vi "Main.vi"(11 "Module Admin":refnum<class "Delacor_lib_QMH_Cloneable Module Admin.lvclass">) -> ()   [LabVIEW 2025, in "My Cloneable Module.lvlib"]
doc: "This template is based off of the Queued Message Handler design pattern and the Queued Message Handler project template that ships with LabVIEW.\n\nThe main difference is that the queue is private to this module and communication between modules is performed via Broadcast and Request events.\n\nRequest events are wrapped in public API methods and are handled in the Event Handling Loop (EHL) of this VI. Any module can register for Broadcast events sent by this module. The EHL generates messages based on user interface actions.\n\nThe Message Handling Loop (MHL) processes messages generated by the EHL, or by other messages. The messages are string values, so new messages can be added easily to the Message Cases case structure in the MHL. Each message cluster can also provide an optional value for Message Data, which is a variant that can be converted to whatever message-specific data is required.\n_____\nBased on DQMH Dev Tools: Project Template 7.1.0.1503."
uses:
  My Cloneable Module.lvlib
  <vilib>/Delacor/Delacor QMH/Libraries/Cloneable Module Admin_class/Delacor_lib_QMH_Cloneable Module Admin.lvclass
  C:/Program Files (x86)/National Instruments/LabVIEW 2025/vi.lib/Delacor/Delacor QMH/Libraries/Module Admin_class/Delacor_lib_QMH_Module Admin.lvclass
  Module Data--cluster.ctl
  Do Something Argument--cluster.ctl
  <vilib>/Delacor/Delacor QMH/Libraries/Cloneable Module Admin_class/Delacor_lib_QMH_Cloneable Module Admin.lvclass/Delacor_lib_QMH_Cloneable Module Admin.ctl
  <vilib>/Delacor/Delacor QMH/Libraries/Message Queue_class/Delacor_lib_QMH_Message Queue.lvclass/Delacor_lib_QMH_Message Queue.ctl
  Do Something Else Argument--cluster.ctl
  Do Something Else and Wait for Reply Argument--cluster.ctl
  Do Something Else and Wait (Reply Payload)--cluster.ctl
  Stop Argument--cluster.ctl
  <vilib>/Delacor/Delacor QMH/Libraries/Module Admin_class/Delacor_lib_QMH_Module Admin.lvclass/Delacor_lib_QMH_Module Admin.ctl
  <vilib>/Utility/miscctls.llb/LVPointTypeDef.ctl
  <vilib>/Delacor/Delacor QMH/Libraries/Message Queue_class/Delacor_lib_QMH_Enqueue Message (Single).vi
  <vilib>/Delacor/Delacor QMH/Libraries/Cloneable Module Admin_class/Delacor_lib_QMH_Get Module ID.vi
  <vilib>/Delacor/Delacor QMH/Libraries/Module Admin_class/Delacor_lib_QMH_Get External Launch.vi
  <vilib>/Delacor/Delacor QMH/Libraries/Message Queue_class/Delacor_lib_QMH_Message Queue.lvclass
panel:
  out "error out":errorcluster
  out "X":dbl
  out "Status":string
  in  "Simulate EHL Error":bool
  in  "Simulate MHL Error":bool
  in  "Do Something Else <Replace Me>":bool
  in  "Do Something <Replace Me>":bool
  # "These controls have associated \"Value Changed\" events configured in the Event Structure on the diagram.\n\nReplace them (and reconfigure the Event Structure) with the controls you need for your application. \n\nOther processes communicate with this Module via its Public API (wrappers for its Request Events).\n\nThis Module communicates with other processes via its Broadcast Events.\nAny process that wants to receive these messages can register for this module's Broadcast events."
  # "This template is for the DQMH framework. See the block diagram for more information on how to use this template."
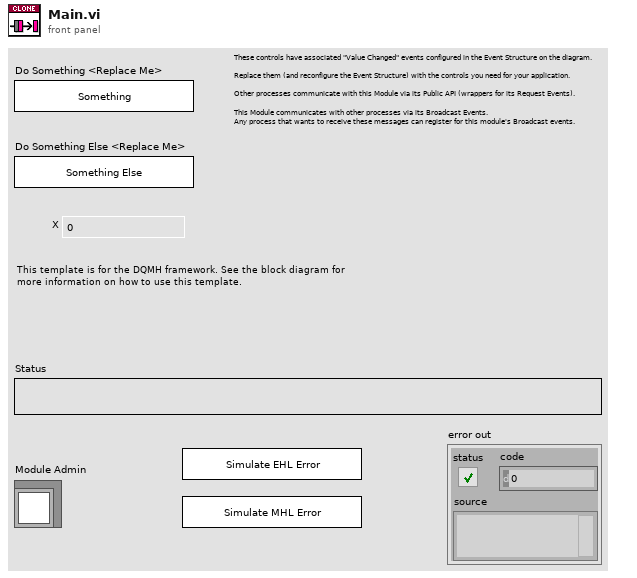
[diagram p1: front panel]
types:
  T1 = typedef "My Cloneable Module.lvlib/Request Events--cluster.ctl" = cluster{"Stop Module":refnum<user-event>, "Do Something":refnum<user-event>, "Do Something Else":refnum<user-event>, "Do Something Else and Wait for Reply":refnum<user-event>, "Show Panel":refnum<user-event>, "Hide Panel":refnum<user-event>, "Show Diagram":refnum<user-event>, "Get Module Execution Status":refnum<user-event>}
  T2 = typedef "My Cloneable Module.lvlib/Module Data--cluster.ctl" = cluster{"Status":string}
  T3 = typedef "My Cloneable Module.lvlib/Do Something Argument--cluster.ctl" = cluster{"Module ID":i32, "Do Something Msg":string}
  T4 = typedef "My Cloneable Module.lvlib/Do Something Else Argument--cluster.ctl" = cluster{"Module ID":i32, "Do Something Else Msg":string, "X":dbl}
  T5 = typedef "My Cloneable Module.lvlib/Do Something Else and Wait for Reply Argument--cluster.ctl" = cluster{"Module ID":i32, "Do Something Else Msg":string, "X":dbl, "Wait Notifier":refnum<notifier>, "wait for reply":bool}
  T6 = enum32{"invalid lock state", "Not Locked", "Locked (No Password)", "Password-protected"}
  T7 = typedef "My Cloneable Module.lvlib/Stop Argument--cluster.ctl" = cluster{"Module ID":i32, "Origin":string, "Exit via Stop Module Req?":bool, "Wait for Module to stop?":bool}
  T8 = typedef "LVPointTypeDef.ctl" = cluster{"Horizontal":i16, "Vertical":i16}
  T9 = enum32{"Invalid", "Standard", "Closed", "Hidden", "Minimized", "Maximized"}
  T10 = typedef "My Cloneable Module.lvlib/Do Something Else and Wait (Reply Payload)--cluster.ctl" = cluster{"Value":dbl, "error":errorcluster, "Module ID":i32}
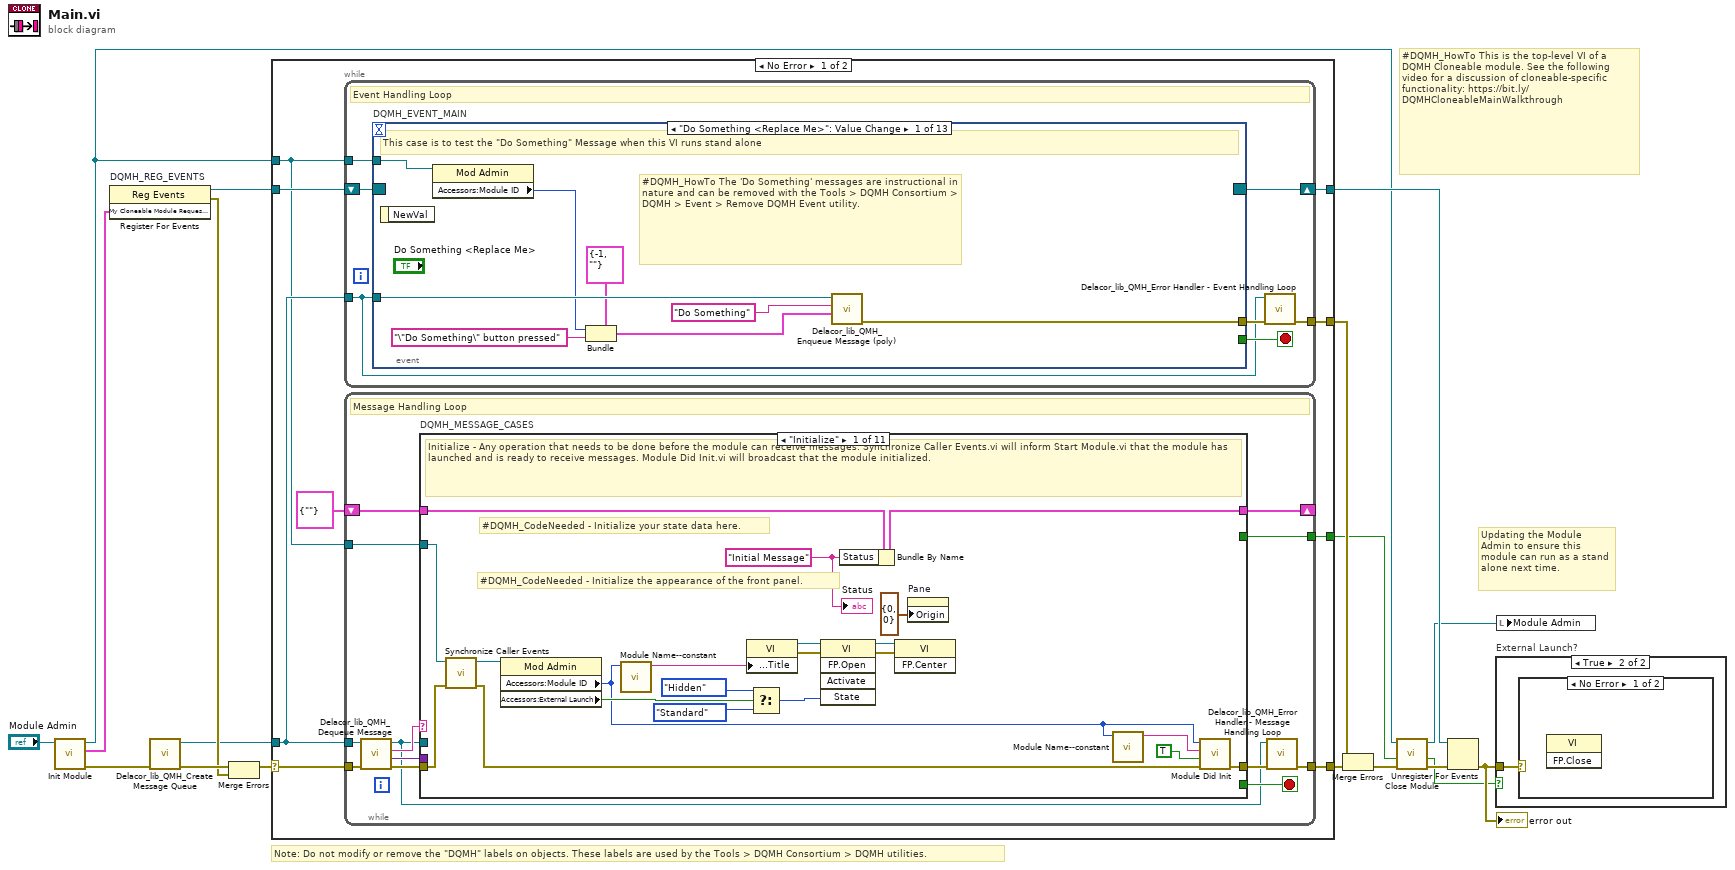
[diagram p0: block diagram]
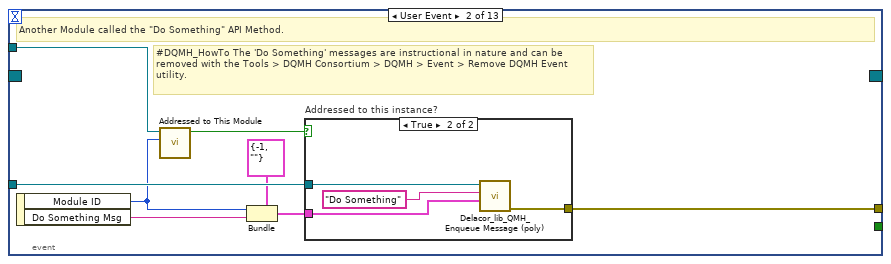
[diagram p2: hidden frame]
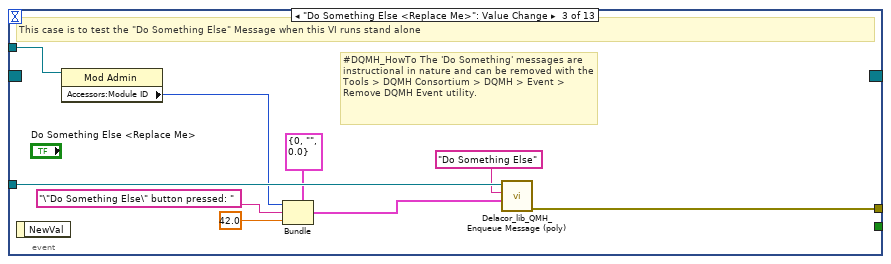
[diagram p4: hidden frame]
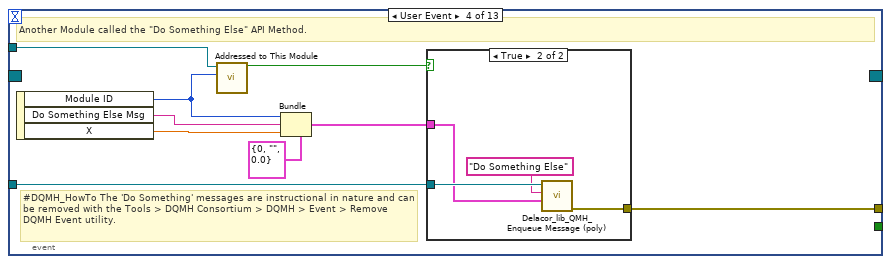
[diagram p5: hidden frame]
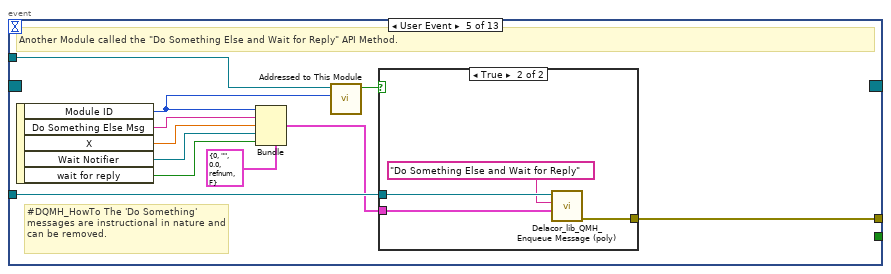
[diagram p7: hidden frame]
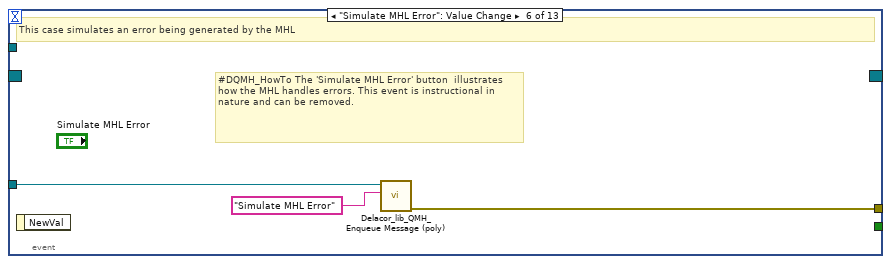
[diagram p9: hidden frame]
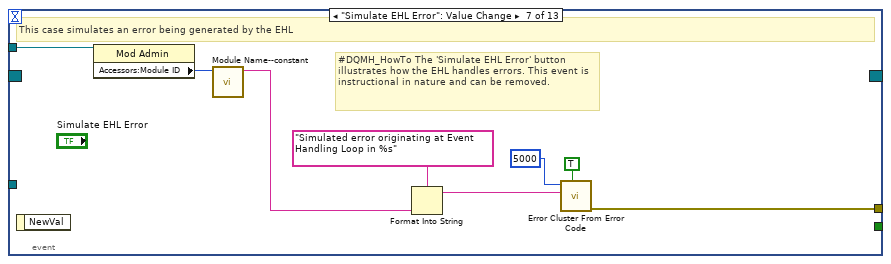
[diagram p10: hidden frame]
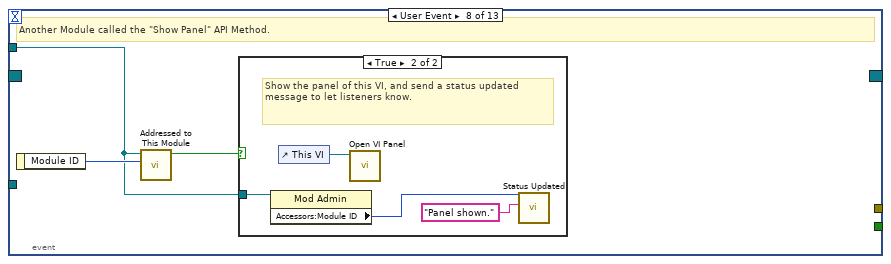
[diagram p11: hidden frame]
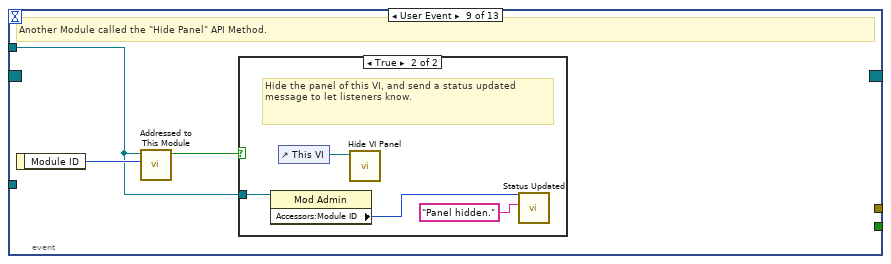
[diagram p13: hidden frame]
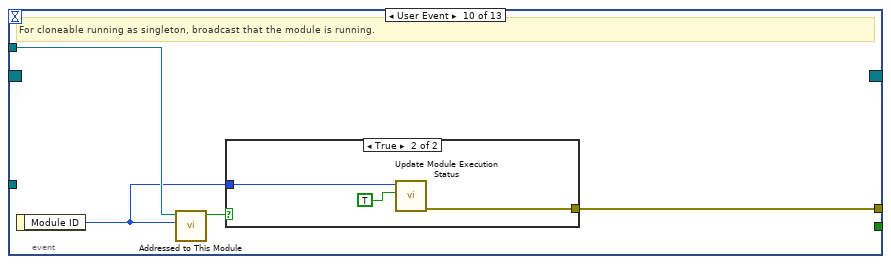
[diagram p15: hidden frame]
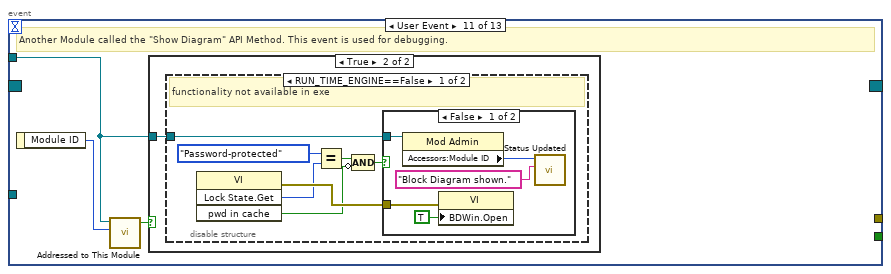
[diagram p17: hidden frame]
diagram:
  # "#DQMH_HowTo This is the top-level VI of a DQMH Cloneable module. See the following video for a discussion of cloneable-specific functionality: https://bit.ly/DQMHCloneableMainWalkthrough"
  # "Note: Do not modify or remove the \"DQMH\" labels on objects. These labels are used by the Tools > DQMH Consortium > DQMH utilities."
  # "Updating the Module Admin to ensure this module can run as a stand alone next time."
  n1 = call "Init Module.vi"("Cloneable Module Admin in"="Module Admin") -> ("error out"=w15:errorcluster, "My Cloneable Module Request Events"=w7:T1, "Cloneable Module Admin out"=w4:refnum<class "Delacor_lib_QMH_Cloneable Module Admin.lvclass">)  [unwired: 8 in]
  n2 = register-events "DQMH_REG_EVENTS"(w7) -> (reference out=w8:refnum<event-registration>, error out=w10:errorcluster)  [unwired: 2 in]
  n3 = call <vilib>:"Delacor_lib_QMH_Create Message Queue.vi"("error in"=w15) -> ("error out"=w12:errorcluster, "Message Queue"=w6:refnum<class "Delacor_lib_QMH_Message Queue.lvclass">)  [unwired: 9 in]
  n4 = Merge Errors(w12, w10) -> (w11:errorcluster)
  n5 = case shown="No Error" w11 {
    selector: w11 -> [w25 w336]
    tunnel: [w27 w335] -> w16
    tunnel: [w24 w334] -> w9
    tunnel: w8 -> [w22 w334]
    tunnel: w6 -> [w21 w327]
    tunnel: [w26 _] -> w17
    tunnel: w4 -> [w20 w330]
    tunnel: [w19 _] -> w2
    frame No Error {
      n6 = while {
        tunnel: w21 -> [w28]
        shift-right: [w31] -> w24
        shift-left: w22 -> [w32]
        tunnel: [w33] -> w26
        tunnel: w20 -> [w29]
        stop <- w30 stop-if-true
        # "Event Handling Loop"
        n7 = event "DQMH_EVENT_MAIN" shown="[0] \"Do Something <Replace Me>\": Value Change" {
          selector: w32 -> [_ _ _ _ _ _ _ _ _ _ _ _ _]
          dyn-events: [_ _ _ _ _ _ _ _ _ _ _ _ _] -> w31
          timeout: _ -> [_ _ _ _ _ _ _ _ _ _ _ _ _]
          tunnel: [_ _ _ _ _ _ _ _ _ _ _ w143 _] -> w30
          tunnel: w28 -> [w41 w49 w62 w71 w86 w93 _ _ _ _ _ w146 w163]
          tunnel: [w42 w50 w63 w72 w87 w94 w102 _ _ w120 _ w147 w166] -> w34
          tunnel: w29 -> [w37 w47 w56 w69 w84 _ w101 w103 w110 w118 w124 w145 w164]
          event "Do Something <Replace Me>": Value Change {
            # "#DQMH_HowTo The 'Do Something' messages are instructional in nature and can be removed with the Tools > DQMH Consortium > DQMH > Event > Remove DQMH Event utility."
            # "This case is to test the \"Do Something\" Message when this VI runs stand alone"
            n8 = event-data() -> ()  [unwired: 1 in, 1 out]
            n9 = property on="Property Node" class="Mod Admin"(reference=w37) -> ("Accessors:Module ID"=w36:i32)  [unwired: 1 in, 2 out]
            n10 = Bundle(cluster=T3 {"Module ID"=-1, "Do Something Msg"=""} ("Do Something Argument"), "Module ID"=w36, "Do Something Msg"="\"Do Something\" button pressed" ("\"Do Something\" button pressed")) -> (w39:T3)
            n11 = call-poly <vilib>:"Delacor_lib_QMH_Enqueue Message (poly).vi"("Message Data"=w39, "Message"="Do Something", "Message Queue in"=w41) -> ("error out"=w42:errorcluster)  [unwired: 7 in, 1 out]
          }
          event User Event {
            # "#DQMH_HowTo The 'Do Something' messages are instructional in nature and can be removed with the Tools > DQMH Consortium > DQMH > Event > Remove DQMH Event utility."
            # "Another Module called the \"Do Something\" API Method."
            n12 = event-data() -> ("Module ID"=w44:i32, "Do Something Msg"=w43:string)  [unwired: 1 in]
            n13 = call "Addressed to This Module.vi"("Module ID from Argument"=w44, "Module Admin"=w47) -> ("Addressed to this instance?"=w48:bool)  [unwired: 8 in, 1 out]
            n14 = Bundle(cluster=T3 {"Module ID"=-1, "Do Something Msg"=""} ("Do Something Argument"), "Module ID"=w44, "Do Something Msg"=w43) -> (w46:T3)
            n15 = case "Addressed to this instance?" shown="True" w48 {
              tunnel: w49 -> [_ w53]
              tunnel: [_ w54] -> w50
              tunnel: w46 -> [_ w51]
              frame False {
                # "Do nothing"
              }
              frame True {
                n16 = call-poly <vilib>:"Delacor_lib_QMH_Enqueue Message (poly).vi"("Message Data"=w51, "Message"="Do Something", "Message Queue in"=w53) -> ("error out"=w54:errorcluster)  [unwired: 7 in, 1 out]
              }
            }
          }
          event "Do Something Else <Replace Me>": Value Change {
            # "#DQMH_HowTo The 'Do Something' messages are instructional in nature and can be removed with the Tools > DQMH Consortium > DQMH > Event > Remove DQMH Event utility."
            # "This case is to test the \"Do Something Else\" Message when this VI runs stand alone"
            n17 = event-data() -> ()  [unwired: 1 in, 1 out]
            n18 = property on="Property Node" class="Mod Admin"(reference=w56) -> ("Accessors:Module ID"=w55:i32)  [unwired: 1 in, 2 out]
            n19 = Bundle(cluster=T4 {"Module ID"=0, "Do Something Else Msg"="", "X"=0.0} ("Do Something Else Argument"), "Module ID"=w55, "Do Something Else Msg"="\"Do Something Else\" button pressed: " ("\"Do Something Else\" button pressed"), "X"=42.0) -> (w59:T4)
            n20 = call-poly <vilib>:"Delacor_lib_QMH_Enqueue Message (poly).vi"("Message Data"=w59, "Message"="Do Something Else", "Message Queue in"=w62) -> ("error out"=w63:errorcluster)  [unwired: 7 in, 1 out]
          }
          event User Event {
            # "#DQMH_HowTo The 'Do Something' messages are instructional in nature and can be removed with the Tools > DQMH Consortium > DQMH > Event > Remove DQMH Event utility."
            # "Another Module called the \"Do Something Else\" API Method."
            n21 = event-data() -> ("Module ID"=w64:i32, "Do Something Else Msg"=w65:string, "X"=w67:dbl)  [unwired: 1 in]
            n22 = call "Addressed to This Module.vi"("Module ID from Argument"=w64, "Module Admin"=w69) -> ("Addressed to this instance?"=w70:bool)  [unwired: 8 in, 1 out]
            n23 = Bundle(cluster=T4 {"Module ID"=0, "Do Something Else Msg"="", "X"=0.0} ("Do Something Else Argument"), "Module ID"=w64, "Do Something Else Msg"=w65, "X"=w67) -> (w66:T4)
            n24 = case shown="True" w70 {
              tunnel: w71 -> [_ w75]
              tunnel: [_ w76] -> w72
              tunnel: w66 -> [_ w73]
              frame False {
              }
              frame True {
                n25 = call-poly <vilib>:"Delacor_lib_QMH_Enqueue Message (poly).vi"("Message Data"=w73, "Message"="Do Something Else", "Message Queue in"=w75) -> ("error out"=w76:errorcluster)  [unwired: 7 in, 1 out]
              }
            }
          }
          event User Event {
            # "#DQMH_HowTo The 'Do Something' messages are instructional in nature and can be removed."
            # "Another Module called the \"Do Something Else and Wait for Reply\" API Method."
            n26 = event-data() -> ("Module ID"=w82:i32, "Do Something Else Msg"=w80:string, "X"=w79:dbl, "Wait Notifier"=w78:refnum<notifier>, "wait for reply"=w77:bool)  [unwired: 1 in]
            n27 = Bundle(cluster=T5 {"Module ID"=0, "Do Something Else Msg"="", "X"=0.0, "Wait Notifier"=refnum, "wait for reply"=FALSE} ("Do Something Else and Wait for Reply Argument"), "Module ID"=w82, "Do Something Else Msg"=w80, "X"=w79, "Wait Notifier"=w78, "wait for reply"=w77) -> (w81:T5)
            n28 = call "Addressed to This Module.vi"("Module ID from Argument"=w82, "Module Admin"=w84) -> ("Addressed to this instance?"=w85:bool)  [unwired: 8 in, 1 out]
            n29 = case shown="True" w85 {
              tunnel: [_ w91] -> w87
              tunnel: w86 -> [_ w90]
              tunnel: w81 -> [_ w88]
              frame False {
              }
              frame True {
                n30 = call-poly <vilib>:"Delacor_lib_QMH_Enqueue Message (poly).vi"("Message Data"=w88, "Message"="Do Something Else and Wait for Reply", "Message Queue in"=w90) -> ("error out"=w91:errorcluster)  [unwired: 7 in, 1 out]
              }
            }
          }
          event "Simulate MHL Error": Value Change {
            # "#DQMH_HowTo The 'Simulate MHL Error' button  illustrates how the MHL handles errors. This event is instructional in nature and can be removed."
            # "This case simulates an error being generated by the MHL"
            n31 = event-data() -> ()  [unwired: 1 in, 1 out]
            n32 = call-poly <vilib>:"Delacor_lib_QMH_Enqueue Message (poly).vi"("Message"="Simulate MHL Error", "Message Queue in"=w93) -> ("error out"=w94:errorcluster)  [unwired: 8 in, 1 out]
          }
          event "Simulate EHL Error": Value Change {
            # "#DQMH_HowTo The 'Simulate EHL Error' button  illustrates how the EHL handles errors. This event is instructional in nature and can be removed."
            # "This case simulates an error being generated by the EHL"
            n33 = event-data() -> ()  [unwired: 1 in, 1 out]
            n34 = property on="Property Node" class="Mod Admin"(reference=w101) -> ("Accessors:Module ID"=w100:i32)  [unwired: 1 in, 2 out]
            n35 = call "Module Name--constant.vi"("Module ID"=w100) -> ("Module Name"=w95:string)  [unwired: 10 in]
            n36 = Format Into String(format string="Simulated error originating at Event Handling Loop in %s", w95) -> (resulting string=w98:string)  [unwired: 2 in, 1 out]
            n37 = call <vilib>:"Error Cluster From Error Code.vi"("show call chain? (False)"=TRUE, "error message (\"\")"=w98, "error code (0)"=5000) -> ("error out"=w102:errorcluster)  [unwired: 6 in]
          }
          event User Event {
            # "Another Module called the \"Show Panel\" API Method."
            n38 = event-data() -> ("Module ID"=w104:i32)  [unwired: 1 in]
            n39 = call "Addressed to This Module.vi"("Module ID from Argument"=w104, "Module Admin"=w103) -> ("Addressed to this instance?"=w105:bool)  [unwired: 8 in, 1 out]
            n40 = case shown="True" w105 {
              tunnel: w103 -> [_ w107]
              frame False {
              }
              frame True {
                # "Show the panel of this VI, and send a status updated message to let listeners know."
                n41 = property on="Property Node" class="Mod Admin"(reference=w107) -> ("Accessors:Module ID"=w106:i32)  [unwired: 1 in, 2 out]
                n42 = control-ref of="This VI"() -> (w109:refnum<vi>)
                n43 = call "Open VI Panel.vi"("VI"=w109) -> ()  [unwired: 10 in, 1 out]
                n44 = call "Status Updated.vi"("Status"="Panel shown." ("format string"), "Module ID"=w106) -> ()  [unwired: 9 in, 1 out]
              }
            }
          }
          event User Event {
            # "Another Module called the \"Hide Panel\" API Method."
            n45 = event-data() -> ("Module ID"=w111:i32)  [unwired: 1 in]
            n46 = call "Addressed to This Module.vi"("Module ID from Argument"=w111, "Module Admin"=w110) -> ("Addressed to this instance?"=w112:bool)  [unwired: 8 in, 1 out]
            n47 = case shown="True" w112 {
              tunnel: w110 -> [_ w114]
              frame False {
              }
              frame True {
                # "Hide the panel of this VI, and send a status updated message to let listeners know."
                n48 = property on="Property Node" class="Mod Admin"(reference=w114) -> ("Accessors:Module ID"=w113:i32)  [unwired: 1 in, 2 out]
                n49 = control-ref of="This VI"() -> (w116:refnum<vi>)
                n50 = call "Hide VI Panel.vi"("VI"=w116) -> ()  [unwired: 10 in, 1 out]
                n51 = call "Status Updated.vi"("Status"="Panel hidden." ("format string"), "Module ID"=w113) -> ()  [unwired: 9 in, 1 out]
              }
            }
          }
          event User Event {
            # "For cloneable running as singleton, broadcast that the module is running."
            n52 = event-data() -> ("Module ID"=w117:i32)  [unwired: 1 in]
            n53 = call "Addressed to This Module.vi"("Module ID from Argument"=w117, "Module Admin"=w118) -> ("Addressed to this instance?"=w119:bool)  [unwired: 8 in, 1 out]
            n54 = case shown="True" w119 {
              tunnel: [_ w123] -> w120
              tunnel: w117 -> [_ w122]
              frame False {
              }
              frame True {
                n55 = call "Update Module Execution Status.vi"("Running?"=TRUE, "Module ID"=w122) -> ("error out"=w123:errorcluster)  [unwired: 9 in]
              }
            }
          }
          event User Event {
            # "Another Module called the \"Show Diagram\" API Method. This event is used for debugging."
            n56 = event-data() -> ("Module ID"=w125:i32)  [unwired: 1 in]
            n57 = call "Addressed to This Module.vi"("Module ID from Argument"=w125, "Module Admin"=w124) -> ("Addressed to this instance?"=w126:bool)  [unwired: 8 in, 1 out]
            n58 = case shown="True" w126 {
              tunnel: w124 -> [_ w127]
              frame False {
              }
              frame True {
                n59 = disable-structure shown="RUN_TIME_ENGINE==False" {
                  disable-tunnel: w127 -> [w128 _]
                  frame condition #0 (active) {
                    # "functionality not available in exe"
                    n60 = invoke on="Invoke Node" class="VI" method="Lock State.Get"() -> (error out=w134:errorcluster, "Get Lock State"=w133:T6, "pwd in cache"=w130:bool)  [unwired: 4 in, 1 out]
                    n61 = Equal?(x=T6."Password-protected", y=w133) -> (x = y?=w131:bool)
                    n62 = Compound Arithmetic op=AND(w131, invert w130) -> (w129:bool)
                    n63 = case shown="False" w129 {
                      tunnel: w134 -> [w139 _]
                      tunnel: w128 -> [w136 _]
                      frame False {
                        n64 = property on="Property Node" class="Mod Admin"(reference=w136) -> ("Accessors:Module ID"=w135:i32)  [unwired: 1 in, 2 out]
                        n65 = property on="Property Node" class="VI"(error in=w139, "BDWin.Open"=TRUE ("Block Diagram Window:Open")) -> ()  [unwired: 1 in, 2 out]
                        n66 = call "Status Updated.vi"("Status"="Block Diagram shown." ("format string"), "Module ID"=w135) -> ()  [unwired: 9 in, 1 out]
                      }
                      frame True {
                        # "Password-protected VI, and the password is not in the cache. Do not show the diagram."
                      }
                    }
                  }
                  frame condition #1 {
                  }
                }
              }
            }
          }
          event User Event {
            # "Another Module called the \"Stop Module\" API Method  or the Message Handling Loop below."
            n67 = event-data() -> ("Module ID"=w141:i32, "Wait for Module to stop?"=w142:bool, "Origin"=w140:string)  [unwired: 1 in]
            n68 = call "Addressed to This Module.vi"("Module ID from Argument"=w141, "Module Admin"=w145) -> ("Addressed to this instance?"=w144:bool)  [unwired: 8 in, 1 out]
            n69 = case shown="True" w144 {
              tunnel: [_ w159] -> w147
              tunnel: w146 -> [_ w155]
              tunnel: [_ TRUE] -> w143
              tunnel: w142 -> [_ w150]
              tunnel: w141 -> [_ w152]
              tunnel: w140 -> [_ w148]
              frame False {
              }
              frame True {
                # "The event can get fired from the Exit message. The queue gets destroyed there. In this case, the Enqueue VI will return error 1. It is safe to ignore, because the module is already exiting."
                n70 = local write "Status"(w148) -> ()
                n71 = Bundle By Name(cluster=T7 {"Module ID"=-1, "Origin"="", "Exit via Stop Module Req?"=FALSE, "Wait for Module to stop?"=FALSE} ("Stop Argument"), "Module ID"=w152, "Exit via Stop Module Req?"=TRUE, "Wait for Module to stop?"=w150) -> (w149:T7)
                n72 = call-poly <vilib>:"Delacor_lib_QMH_Enqueue Message (poly).vi"("Priority Message? (F)"=TRUE, "Message Data"=w149, "Message"="Exit", "Message Queue in"=w155) -> ("error out"=w160:errorcluster)  [unwired: 6 in, 1 out]
                n73 = call <vilib>:"Clear Errors.vi"("error in (no error)"=w160, "specific error code to clear (0: all)"=1) -> ("error out"=w159:errorcluster)  [unwired: 4 in, 1 out]
              }
            }
          }
          event Panel Close? {
            w165 = TRUE  # Discard the event, the MHL is responsible for closing and stopping this VI.
            # "Hide the panel or send the 'Exit' message if the user clicks the 'X' on the module main VI panel."
            n74 = event-data() -> ()  [unwired: 1 in, 1 out]
            n75 = property on="Property Node" class="Mod Admin"(reference=w164) -> (reference out=w161:refnum<class "Delacor_lib_QMH_Cloneable Module Admin.lvclass">, "Accessors:External Launch"=w162:bool)  [unwired: 1 in, 1 out]
            n76 = case shown="True" w162 {
              tunnel: w163 -> [_ w174]
              tunnel: [_ w175] -> w166
              tunnel: w161 -> [w169 _]
              frame True {
                # "If externally launched, clicking the 'X' hides the panel, but doesn't close it."
                n77 = property on="Property Node" class="Mod Admin"(reference=w169) -> ("Accessors:Module ID"=w168:i32)  [unwired: 1 in, 2 out]
                n78 = call "Status Updated.vi"("Status"="Panel hidden." ("format string"), "Module ID"=w168) -> ("error out"=w167:errorcluster)  [unwired: 9 in]
                n79 = control-ref of="This VI"() -> (w171:refnum<vi>)
                n80 = call "Hide VI Panel.vi"("error in"=w167, "VI"=w171) -> ()  [unwired: 9 in, 1 out]
              }
              frame False {
                # "If run as a stand-alone VI, clicking the panel 'X' stops the VI."
                n81 = call-poly <vilib>:"Delacor_lib_QMH_Enqueue Message (poly).vi"("Priority Message? (F)"=TRUE, "Message"="Exit", "Message Queue in"=w174) -> ("error out"=w175:errorcluster)  [unwired: 7 in, 1 out]
              }
            }
            n82 = event-data ("Event Filter Node")("Discard?"=w165) -> ()  [unwired: 1 in, 1 out]
          }
        }
        n83 = call-dynamic "Delacor_lib_QMH_Error Handler - Event Handling Loop.vi"("error in"=w34, "Message Queue in"=w28) -> ("dup error in"=w33:errorcluster)  [unwired: 8 in, 1 out]
      }
      n84 = while {
        tunnel: w21 -> [w176]
        shift-right: [w183] -> _
        shift-left: T2 {"Status"=""} ("Data Cluster") -> [w184]
        tunnel: w25 -> [w187]
        tunnel: [w185] -> w27
        tunnel: w20 -> [w178]
        tunnel: [w177] -> w19
        stop <- w182 stop-if-true
        # "Message Handling Loop"
        n85 = call-dynamic "Delacor_lib_QMH_Dequeue Message.vi"("error in"=w187, "Message Queue in"=w176) -> ("error out"=w186:errorcluster, "Message Data"=w180:variant, "Message"=w181:string, "Message Queue out"=w179:refnum<class "Delacor_lib_QMH_Message Queue.lvclass">)  [unwired: 6 in]
        n86 = case "DQMH_MESSAGE_CASES" shown="\"Initialize\"" w181 {
          selector: w181 -> [_ _ _ _ _ _ _ _ _ _ w316]
          tunnel: w179 -> [_ _ _ _ _ _ _ w271 _ w308 _]
          tunnel: w186 -> [w207 w211 w221 w232 w253 w266 w268 w280 w297 w314 w325]
          tunnel: [w205 w211 w219 w231 w252 w265 w268 w276 w296 w309 w326] -> w188
          tunnel: w184 -> [w198 w210 w218 w230 w233 w264 w267 w275 w294 w307 w323]
          tunnel: [w197 w210 w218 w230 w233 w264 w267 w275 w294 w307 w323] -> w183
          tunnel: [_ _ _ _ _ _ _ _ _ w306 _] -> w182
          tunnel: w180 -> [_ _ w217 w227 w247 _ _ w274 _ w304 _]
          tunnel: w178 -> [w193 _ w213 w223 w238 _ _ w273 w292 w299 w322]
          tunnel: [_ _ _ _ _ _ _ _ _ w302 _] -> w177
          frame "Initialize" {
            w190 = "Initial Message" ("Initial Message")
            # "#DQMH_CodeNeeded - Initialize the appearance of the front panel."
            # "#DQMH_CodeNeeded - Initialize your state data here."
            # "Initialize - Any operation that needs to be done before the module can receive messages. Synchronize Caller Events.vi will inform Start Module.vi that the module has launched and is ready to receive messages. Module Did Init.vi will broadcast that the module initialized."
            n87 = call "Synchronize Caller Events.vi"("error in"=w207, "Module Admin"=w193) -> ("error out"=w206:errorcluster, "Module Admin out"=w192:refnum<class "Delacor_lib_QMH_Cloneable Module Admin.lvclass">)  [unwired: 8 in]
            n88 = property on="Property Node" class="Mod Admin"(reference=w192) -> ("Accessors:Module ID"=w189:i32, "Accessors:External Launch"=w194:bool)  [unwired: 1 in, 2 out]
            n89 = call "Module Name--constant.vi"("Module ID"=w189) -> ("Module Name"=w202:string)  [unwired: 10 in]
            n90 = property on="Property Node" class="VI"("Front Panel.Title"=w202) -> (reference out=w204:refnum<vi>, error out=w209:errorcluster)  [unwired: 2 in]
            n91 = Select(t=T9."Hidden" ("State"), s=w194, f=T9."Standard" ("State")) -> (s? t:f=w199:T9)
            n92 = invoke on="Invoke Node" class="VI" method="FP.Open"(reference=w204, error in=w209, "State"=w199) -> (reference out=w203:refnum<vi>, error out=w208:errorcluster)  [unwired: 2 in, 3 out]
            n93 = Bundle By Name(cluster=w198, "Status"=w190) -> (w197:T2)
            n94 = invoke on="Invoke Node" class="VI" method="FP.Center"(reference=w203, error in=w208) -> ()  [unwired: 1 in, 3 out]
            n95 = property on="Pane" class="Pane"("Origin"=T8 {"Horizontal"=0, "Vertical"=0}) -> ()  [unwired: 2 in, 2 out]
            n96 = call "Module Name--constant.vi"("Module ID"=w189) -> ("Module Name"=w195:string)  [unwired: 10 in]
            n97 = call "Module Did Init.vi"("error in"=w206, "Initialized?"=TRUE, "Origin"=w195, "Module ID"=w189) -> ("error out"=w205:errorcluster)  [unwired: 7 in]
            "Status" <- w190
          }
          frame "---Module Specific---" {
            # "Separator -- The following cases handle messages specific to this Module."
          }
          frame "Do Something" {
            # "#DQMH_HowTo The 'Do Something' messages are instructional in nature and can be removed with the Tools > DQMH Consortium > DQMH > Event > Remove DQMH Event utility."
            # "Do Something - Replace this message with functionality for your own application. Note that this message also fires the \"Did Something\" broadcast event."
            n98 = Variant To Data(error in=w221, type=T3 {"Module ID"=-1, "Do Something Msg"=""} ("Do Something Argument"), Variant=w217) -> (data=w216:T3, error out=w220:errorcluster)
            n99 = property on="Property Node" class="Mod Admin"(reference=w213) -> ("Accessors:Module ID"=w212:i32)  [unwired: 1 in, 2 out]
            n100 = Unbundle By Name(w216) -> ("Do Something Msg"=w214:string)
            n101 = call "Status Updated.vi"("Status"=w214, "Module ID"=w212) -> ()  [unwired: 9 in, 1 out]
            n102 = local write "Status"(w214) -> ()
            n103 = call "Did Something.vi"("error in"=w220, "Did Something Msg"=w214, "Module ID"=w212) -> ("error out"=w219:errorcluster)  [unwired: 8 in]
          }
          frame "Do Something Else" {
            # "#DQMH_HowTo The 'Do Something' messages are instructional in nature and can be removed with the Tools > DQMH Consortium > DQMH > Event > Remove DQMH Event utility."
            # "Do Something Else - Replace this message with functionality for your own application."
            n104 = Variant To Data(error in=w232, type=T4 {"Module ID"=0, "Do Something Else Msg"="", "X"=0.0} ("Do Something Else Argument"), Variant=w227) -> (data=w228:T4, error out=w231:errorcluster)
            n105 = Unbundle By Name(w228) -> ("Do Something Else Msg"=w226:string, "X"=w225:dbl)
            "X" <- w225
            n106 = property on="Property Node" class="Mod Admin"(reference=w223) -> ("Accessors:Module ID"=w222:i32)  [unwired: 1 in, 2 out]
            n107 = Format Into String(initial string=w226, w225) -> (resulting string=w224:string)  [unwired: 2 in, 1 out]
            n108 = call "Status Updated.vi"("Status"=w224, "Module ID"=w222) -> ()  [unwired: 9 in, 1 out]
            n109 = local write "Status"(w224) -> ()
          }
          frame "Do Something Else and Wait for Reply" {
            w240 = "X(%.2f)+Offset(%.2f)=%.2f"  # status message format string
            # "#DQMH_HowTo The 'Do Something' messages are instructional in nature and can be removed."
            # "Send back X with a random offset"
            # "Do Something Else and Wait for Reply - Replace this message with functionality for your own application. Note that this message must fire a notifier to let callers know it has finished execution, and it returns an error if the 'Value' is negative."
            n110 = property on="Property Node" class="Mod Admin"(reference=w238) -> ("Accessors:Module ID"=w235:i32)  [unwired: 1 in, 2 out]
            n111 = Variant To Data(error in=w253, type=T5 {"Module ID"=0, "Do Something Else Msg"="", "X"=0.0, "Wait Notifier"=refnum, "wait for reply"=FALSE} ("Do Something Else and Wait for Reply Argument"), Variant=w247) -> (data=w248:T5, error out=w251:errorcluster)
            n112 = Unbundle By Name(w248) -> ("Wait Notifier"=w245:refnum<notifier>, "Do Something Else Msg"=w246:string, "X"=w242:dbl, "wait for reply"=w236:bool)
            n113 = Random Number (0-1)() -> (number: 0 to 1=w241:dbl)
            n114 = Add(x=w241, y=w242) -> (x+y=w237:dbl)
            n115 = Less Than 0?(x=w237) -> (x < 0?=w234:bool)
            n116 = local write "X"(w242) -> ()
            n117 = case shown="True" w234 {
              tunnel: [_ w257] -> w250
              frame False {
              }
              frame True {
                n118 = call <vilib>:"Error Cluster From Error Code.vi"("show call chain? (False)"=TRUE, "error message (\"\")"="The 'Something Else and Wait for Reply' message generated a negative number, which is considered an error condition.", "error code (0)"=5000) -> ("error out"=w257:errorcluster)  [unwired: 6 in]
              }
            }
            n119 = Format Into String(format string=w240, initial string=w246, w242, w241, w237) -> (resulting string=w239:string)  [unwired: 1 in, 1 out]
            n120 = Bundle By Name(cluster=T10 {"Value"=0.0, "error"={"status"=FALSE, "code"=0, "source"=""}, "Module ID"=0} ("notification"), "error"=w250, "Value"=w237, "Module ID"=w235) -> (w243:T10)
            n121 = call "Status Updated.vi"("Status"=w239, "Module ID"=w235) -> ()  [unwired: 9 in, 1 out]
            n122 = local write "Status"(w239) -> ()
            n123 = case shown="True" w236 {
              tunnel: w245 -> [_ w261]
              tunnel: w243 -> [_ w260]
              frame False {
              }
              frame True {
                # "Simulate an operation that requires a wait."
                n124 = flat-sequence {
                  tunnel: w261 -> [w263]
                  tunnel: w260 -> [w262]
                  tunnel: w258 -> [_]
                  frame #0 {
                    n125 = Send Notification(notification=w262, notifier=w263) -> ()  [unwired: 1 in, 2 out]
                  }
                }
                n126 = Wait (ms)(milliseconds to wait=u32 1000) -> (millisecond timer value=w258:u32)
              }
            }
            n127 = Merge Errors(w251, w250) -> (w252:errorcluster)
          }
          frame "---Copy This Frame---" {
            # "Duplicate this frame when creating new messages.  Change this comment in the duplicated frame to describe this message."
            n128 = Merge Errors(w266) -> (w265:errorcluster)
          }
          frame "---Exit and Error Handling---" {
            # "Separator - the following cases handle errors and exit messages."
          }
          frame "Error" {
            # "#DQMH_CodeRecommended - If the module is running in standalone mode (External Launch = FALSE), this code will pop up an error dialog and call the 'Exit' message if an error occurs. Add more fine-grained error management here."
            # "Error - Check the error message data and respond accordingly. This message is sent by the \"Error Handler\" VIs at the end of each loop in this application."
            n129 = property on="Property Node" class="Mod Admin"(reference=w273) -> ("Accessors:External Launch"=w272:bool, "Accessors:Module ID"=w270:i32)  [unwired: 1 in, 2 out]
            n130 = Variant To Data(error in=w280, type=errorcluster {"status"=FALSE, "code"=0, "source"=""} ("error constant"), Variant=w274) -> (data=w269:errorcluster, error out=w278:errorcluster)
            n131 = local write "error out"(w269) -> ()
            n132 = call "Error Reported.vi"("Error"=w269, "Module ID"=w270) -> ()  [unwired: 9 in, 1 out]
            n133 = case shown="False" w272 {
              tunnel: [w285 _] -> w277
              tunnel: w271 -> [w283 _]
              tunnel: w269 -> [w284 _]
              frame False {
                n134 = disable-structure shown="Default" {
                  disable-tunnel: w284 -> [w286 _]
                  frame condition #0 (active) {
                    # "If the module is running standalone, then pop up an error dialog and call the \"Exit\" message."
                    n135 = call <vilib>:"Simple Error Handler.vi"("error in (no error)"=w286) -> ()  [unwired: 4 in, 5 out]
                  }
                  frame condition #1 {
                    # "To prevent the Simple Error Handler VI from being loaded (e.g. when deploying to a Real-Time target), add the Conditional Disable Symbol \"DQMH_Disable_SEH\" to your project and set it to TRUE."
                  }
                }
                n136 = call-poly <vilib>:"Delacor_lib_QMH_Enqueue Message (poly).vi"("Priority Message? (F)"=TRUE, "Message"="Exit", "Message Queue in"=w283) -> ("error out"=w285:errorcluster)  [unwired: 7 in, 1 out]
              }
              frame True {
                # "If the module was launched externally, calling the Error Reported broadcast VI is the only action performed by the \"Error\" message. The module's caller can then process the error appropriately."
              }
            }
            n137 = Merge Errors(w278, w277) -> (w276:errorcluster)
          }
          frame "Simulate MHL Error" {
            # "#DQMH_HowTo The 'Simulate MHL Error' button  illustrates how the MHL handles errors. This event is instructional in nature and can be removed."
            # "Simulate an error occurring at the MHL"
            n138 = property on="Property Node" class="Mod Admin"(reference=w292) -> ("Accessors:Module ID"=w293:i32)  [unwired: 1 in, 2 out]
            n139 = call "Module Name--constant.vi"("Module ID"=w293) -> ("Module Name"=w288:string)  [unwired: 10 in]
            n140 = Format Into String(format string="Simulated error originating at Message Handling Loop in %s", w288) -> (resulting string=w289:string)  [unwired: 2 in, 1 out]
            n141 = call <vilib>:"Error Cluster From Error Code.vi"("show call chain? (False)"=TRUE, "error message (\"\")"=w289, "error code (0)"=5001) -> ("error out"=w295:errorcluster)  [unwired: 6 in]
            n142 = Merge Errors(w297, w295) -> (w296:errorcluster)
          }
          frame "Exit" {
            w305 = 91  # 91: not all Exit messages will have an argument
            w306 = TRUE  # Stop the VI
            # "Release the message queue reference"
            # "#DQMH_CodeNeeded - Add any required cleanup code here."
            # "Exit - Exit the application."
            n143 = Variant To Data(error in=w314, type=T7 {"Module ID"=-1, "Origin"="", "Exit via Stop Module Req?"=FALSE, "Wait for Module to stop?"=FALSE} ("Stop Argument"), Variant=w304) -> (data=w301:T7, error out=w310:errorcluster)
            n144 = call <vilib>:"Clear Errors.vi"("error in (no error)"=w310, "specific error code to clear (0: all)"=w305) -> ("error out"=w313:errorcluster)  [unwired: 4 in, 1 out]
            n145 = property on="Property Node" class="Mod Admin"(reference=w299) -> ("Accessors:Module ID"=w298:i32)  [unwired: 1 in, 2 out]
            n146 = control-ref of="This VI"() -> (w300:refnum<vi>)
            n147 = call-dynamic "Delacor_lib_QMH_Release Message Queue.vi"("error in"=w313, "Message Queue"=w308) -> ("error out"=w312:errorcluster)  [unwired: 9 in]
            n148 = call "Handle Exit.vi"("Stop Argument"=w301, "Module Admin in"=w299, "VI reference"=w300) -> ("error out"=w311:errorcluster, "Wait for Stop?"=w302:bool)  [unwired: 7 in]
            n149 = Merge Errors(w312, w311) -> (w309:errorcluster)
            n150 = call "Error Reported.vi"("Error"=w309, "Module ID"=w298) -> ()  [unwired: 9 in, 1 out]
          }
          frame Default {
            # "'Default' case only runs if there is a message that isn't defined in any of the other cases.  Output a programming error."
            n151 = property on="Property Node" class="Mod Admin"(reference=w322) -> ("Accessors:Module ID"=w321:i32)  [unwired: 1 in, 2 out]
            n152 = call "Module Name--constant.vi"("Module ID"=w321) -> ("Module Name"=w315:string)  [unwired: 10 in]
            n153 = Format Into String(format string="The invalid message string \"%s\" was received in the Message Handling Loop for module \"%s\".", w316, w315) -> (resulting string=w318:string)  [unwired: 2 in, 1 out]
            n154 = call <vilib>:"Error Cluster From Error Code.vi"("show call chain? (False)"=TRUE, "error message (\"\")"=w318, "error code (0)"=1) -> ("error out"=w324:errorcluster)  [unwired: 6 in]
            n155 = Merge Errors(w325, w324) -> (w326:errorcluster)
          }
        }
        n156 = call-dynamic "Delacor_lib_QMH_Error Handler - Message Handling Loop.vi"("error in"=w188, "Message Queue in"=w179) -> ("dup error in"=w185:errorcluster)  [unwired: 8 in, 1 out]
      }
    }
    frame Error {
      n157 = call "Synchronize Caller Events.vi"("Module Admin"=w330) -> ("Module Admin out"=w329:refnum<class "Delacor_lib_QMH_Cloneable Module Admin.lvclass">)  [unwired: 9 in, 1 out]
      n158 = property on="Property Node" class="Mod Admin"(reference=w329) -> ("Accessors:Module ID"=w328:i32)  [unwired: 1 in, 2 out]
      n159 = call-dynamic "Delacor_lib_QMH_Release Message Queue.vi"("error in"=w336, "Message Queue"=w327) -> ("error out"=w335:errorcluster)  [unwired: 9 in]
      n160 = call "Module Name--constant.vi"("Module ID"=w328) -> ("Module Name"=w333:string)  [unwired: 10 in]
      n161 = Format Into String(format string="An error occurred during initialization. %s is no longer running.", w333) -> (resulting string=w331:string)  [unwired: 2 in, 1 out]
      n162 = call "Error Reported.vi"("Additional Information"=w331, "Error"=w335, "Module ID"=w328) -> ()  [unwired: 8 in, 1 out]
    }
  }
  n163 = Merge Errors(w17, w16) -> (w18:errorcluster)
  n164 = call "Close Module.vi"("error in"=w18, "Wait for stop?"=w2, "Module Admin in"=w4) -> ("error out"=w14:errorcluster, "External Launch"=w1:bool, "Module Admin out"=w3:refnum<class "Delacor_lib_QMH_Cloneable Module Admin.lvclass">)  [unwired: 6 in]
  n165 = Unregister For Events(event registration refnum=w9, error in=w14) -> (error out=w13:errorcluster)
  "error out" <- w13
  n166 = case "External Launch?" shown="True" w1 {
    tunnel: w13 -> [_ w337]
    frame False {
    }
    frame True {
      n167 = case shown="No Error" w337 {
        frame No Error {
          n168 = invoke class="VI" method="FP.Close"() -> ()  [unwired: 3 in, 3 out]
        }
        frame Error {
          n169 = disable-structure shown="Default" {
            frame condition #0 (active) {
              n170 = invoke class="VI" method="FP.Open"("Activate"=TRUE ("Activate?")) -> ()  [unwired: 4 in, 5 out]
            }
            frame condition #1 {
              # "Don't show panel on error if running inside a built EXE."
            }
          }
        }
      }
    }
  }
  n171 = local write "Module Admin"(w3) -> ()
